vi "Rect-4C to CenterSize or StartEnd.vi"(8 "Image size":T1, 11 "Rect-4C":T4) -> (0 "CenterSize":T2, 3 "StartEnd":T3)   [LabVIEW 2012]
uses:
  <vilib>/Utility/miscctls.llb/LVBoundsTypeDef.ctl
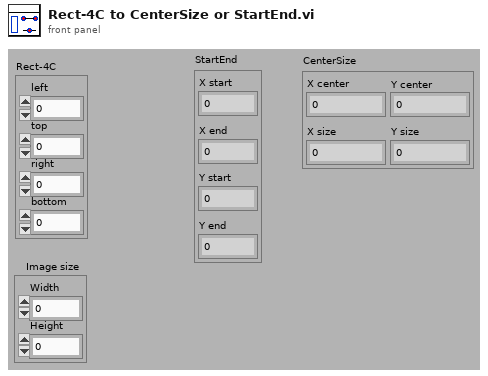
[diagram p1: front panel]
types:
  T1 = typedef "LVBoundsTypeDef.ctl" = cluster{"Width":u32, "Height":u32}
  T2 = cluster{"X center":dbl, "Y center":dbl, "X size":dbl, "Y size":dbl}
  T3 = cluster{"X start":dbl, "X end":dbl, "Y start":dbl, "Y end":dbl}
  T4 = cluster{"left":i16, "top":i16, "right":i16, "bottom":i16}
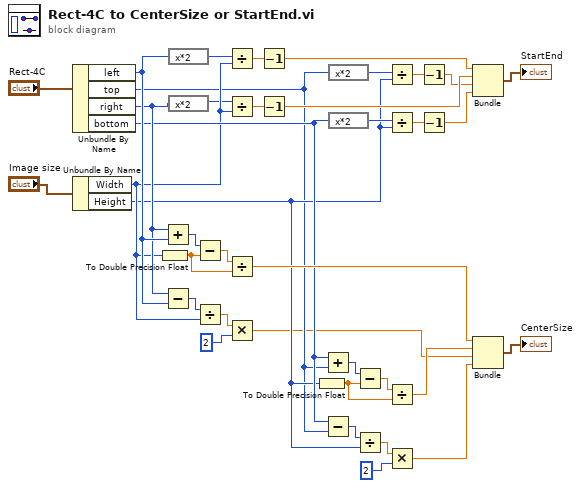
[diagram p0: block diagram]
diagram:
  n1 = Unbundle By Name("Rect-4C") -> ("left"=w21:i16, "top"=w6:i16, "right"=w11:i16, "bottom"=w10:i16)
  n2 = Unbundle By Name("Image size") -> ("Width"=w9:u32, "Height"=w7:u32)
  n3 = To Double Precision Float(number=w9) -> (double precision float=w4:dbl)
  n4 = Add(x=w11, y=w21) -> (x+y=w25:i16)
  n5 = Subtract(x=w11, y=w21) -> (x-y=w22:i16)
  n6 = expression code="x*2"(w21) -> (w37:i16)
  n7 = expression code="x*2"(w11) -> (w8:i16)
  n8 = Subtract(x=w25, y=w4) -> (x-y=w24:dbl)
  n9 = Divide(x=w22, y=w9) -> (x/y=w19:dbl)
  n10 = Divide(x=w37, y=w9) -> (x/y=w36:dbl)
  n11 = Divide(x=w8, y=w9) -> (x/y=w35:dbl)
  n12 = Divide(x=w24, y=w4) -> (x/y=w23:dbl)
  n13 = Multiply(x=w19, y=i16 2) -> (x*y=w1:dbl)
  n14 = Decrement(x=w36) -> (x-1=w30:dbl)
  n15 = Decrement(x=w35) -> (x-1=w29:dbl)
  n16 = To Double Precision Float(number=w7) -> (double precision float=w3:dbl)
  n17 = Add(x=w10, y=w6) -> (x+y=w14:i16)
  n18 = Subtract(x=w10, y=w6) -> (x-y=w16:i16)
  n19 = expression code="x*2"(w6) -> (w31:i16)
  n20 = expression code="x*2"(w10) -> (w34:i16)
  n21 = Subtract(x=w14, y=w3) -> (x-y=w15:dbl)
  n22 = Divide(x=w16, y=w7) -> (x/y=w18:dbl)
  n23 = Divide(x=w31, y=w7) -> (x/y=w32:dbl)
  n24 = Divide(x=w34, y=w7) -> (x/y=w33:dbl)
  n25 = Divide(x=w15, y=w3) -> (x/y=w2:dbl)
  n26 = Multiply(x=w18, y=i16 2) -> (x*y=w13:dbl)
  n27 = Decrement(x=w32) -> (x-1=w28:dbl)
  n28 = Decrement(x=w33) -> (x-1=w27:dbl)
  n29 = Bundle(w30, w29, w28, w27) -> (→"StartEnd":cluster{dbl, dbl, dbl, dbl})  [unwired: 1 in]
  n30 = Bundle(w23, w2, w1, w13) -> (→"CenterSize":cluster{dbl, dbl, dbl, dbl})  [unwired: 1 in]
